vi "ULS Mightex Buffered CCD.vi"(8 "error in (no error)":errorcluster, 9 "Setting Para(RAW)":T1={"Gain"=6, "Sharpness"=0, "Gamma"=1, "CCD Frequemcy"=0, "Brightness"=0, "Contrast"=0}, 10 "Exposure time(RAW)":u32, 11 "IFD in":refnum<class "IFD.lvclass">) -> (0 "error out":errorcluster, 3 "IFD out":refnum<class "IFD.lvclass">)   [LabVIEW 2016, in "IFD.lvclass"]
uses:
  IFD.lvclass
  Tag/IFD_Tag.lvclass/IFD_Tag.ctl
  IFD.lvclass/IFD.ctl
  Tag/IFD_Tag.lvclass
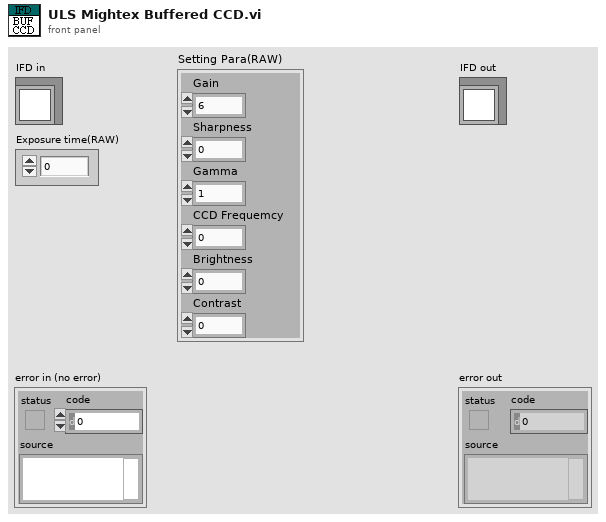
[diagram p1: front panel]
types:
  T1 = cluster{"Gain":u8, "Sharpness":u8, "Gamma":u8, "CCD Frequemcy":u8, "Brightness":u16, "Contrast":u16}
  T2 = enum16{"Undefined(DO NOT USE)", "U8", "ASCII", "U16", "U32", "RATIONAL", "I8", "Undefined 8 bit", "I16", "I32", "SRATIONAL", "SGL", "DBL"}
  T3 = cluster{"Gain":u8, "Sharpness":u8, "Gamma":u8, "CCD Frequemcy":u8}
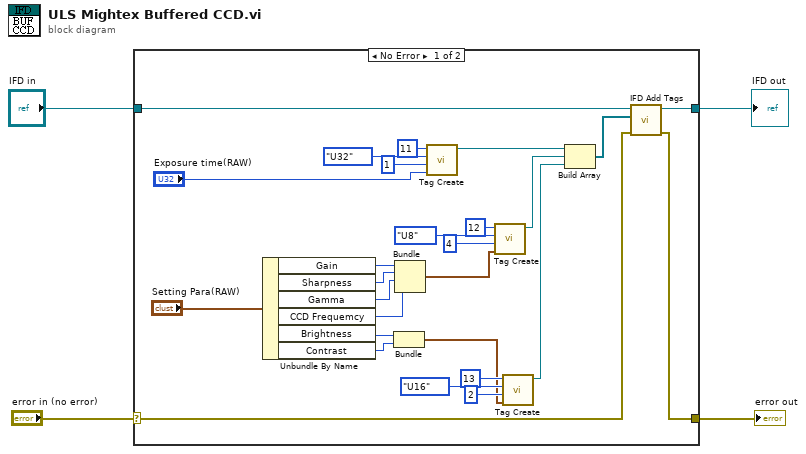
[diagram p0: block diagram]
diagram:
  n1 = case shown="No Error" "error in (no error)" {
    selector: "error in (no error)" -> [w31 w33]
    tunnel: [w30 w33] -> w3
    tunnel: [w29 w32] -> w1
    tunnel: "IFD in" -> [w28 w32]
    frame No Error {
      n2 = Unbundle By Name("Setting Para(RAW)") -> ("Gain"=w20:u8, "Sharpness"=w19:u8, "Gamma"=w18:u8, "CCD Frequemcy"=w17:u8, "Brightness"=w16:u16, "Contrast"=w15:u16)
      n3 = Bundle("Brightness"=w16, "Contrast"=w15) -> (w6:cluster{"Brightness":u16, "Contrast":u16})  [unwired: 1 in]
      n4 = Bundle("Gain"=w20, "Sharpness"=w19, "Gamma"=w18, "CCD Frequemcy"=w17) -> (w11:T3)  [unwired: 1 in]
      n5 = call "Tag Create.vi"("Data"="Exposure time(RAW)", "Data Count"=u32 1, "Data Type"=T2."U32", "Tag ID"=u16 11) -> ("IFD_Tag out"=w22:refnum<class "IFD_Tag.lvclass">)  [unwired: 7 in]
      n6 = call "Tag Create.vi"("Data"=w11, "Data Count"=u32 4, "Data Type"=T2."U8", "Tag ID"=u16 12) -> ("IFD_Tag out"=w10:refnum<class "IFD_Tag.lvclass">)  [unwired: 7 in]
      n7 = call "Tag Create.vi"("Data"=w6, "Data Count"=u32 2, "Data Type"=T2."U16", "Tag ID"=u16 13) -> ("IFD_Tag out"=w5:refnum<class "IFD_Tag.lvclass">)  [unwired: 7 in]
      n8 = Build Array(w22, w10, w5) -> (w23:refnum<class "IFD_Tag.lvclass">[])
      n9 = call "IFD Add Tags.vi"("error in (no error)"=w31, "Tag(s)"=w23, "IFD in"=w28) -> ("error out"=w30:errorcluster, "IFD out"=w29:refnum<class "IFD.lvclass">)  [unwired: 7 in]
    }
    frame Error {
    }
  }
  "error out" <- w3
  "IFD out" <- w1
